vi "Test All.vi"(11 "Error in":errorcluster) -> (15 "Error out":errorcluster)   [LabVIEW 2020, in "CelsiusToFarenheitTests.lvlib"]
doc: "This vi runs all the test cases for the Celsius to Fahrenheit assignment. Also the test report gets saved as a xml format.\n\n* USES *\nDrona, G-CLI and Caraya"
uses:
  CelsiusToFarenheitTests.lvlib
  <vilib>/addons/_JKI Toolkits/Caraya/classes/Test Suite/Define Test Suite (JUnit Report).vi
  <vilib>/Utility/error.llb/Error Cluster From Error Code.vi
  <vilib>/ErrorRing/Error Ring.xnode
  <vilib>/addons/_JKI Toolkits/Caraya/classes/Test Suite/Test Suite.lvclass
  <vilib>/addons/_JKI Toolkits/Caraya/classes/Test/Test.lvclass
  <vilib>/Wiresmith Technology/G CLI/CLI Class/CLI.lvclass
panel:
  # "TESTING ALL TEST CASES FOR CELSIUS TO FAHRENHEIT"
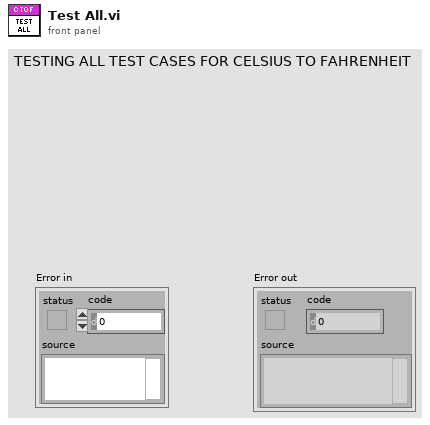
[diagram p1: front panel]
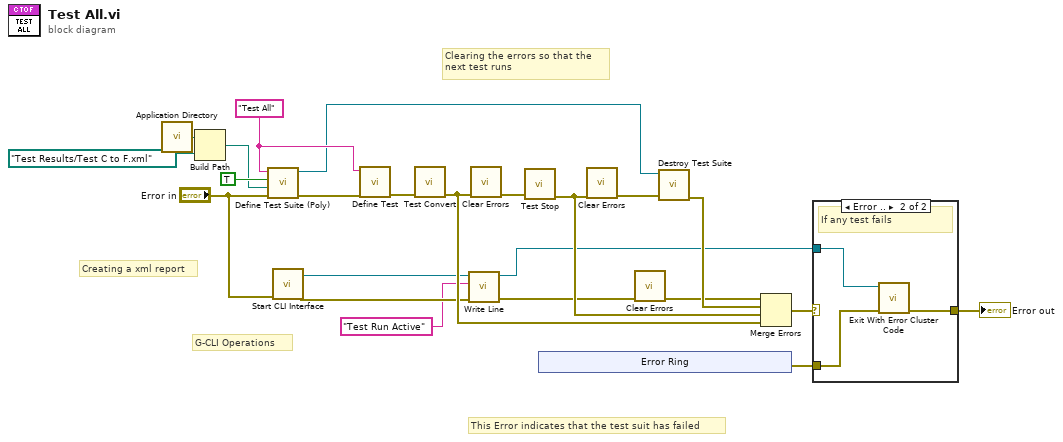
[diagram p0: block diagram]
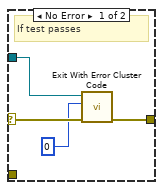
[diagram p2: hidden frame]
diagram:
  w18 = "Test All" ("Label (VI Title)")
  # "This Error indicates that the test suit has failed"
  # "G-CLI Operations"
  # "Creating a xml report"
  # "Clearing the errors so that the\nnext test runs"
  n1 = call <vilib>:"Application Directory.vi"() -> ("Application Directory"=w23:path)
  n2 = Build Path(base path=w23, name or relative path=path "Test Results/Test C to F.xml") -> (appended path=w20:path)
  n3 = call-poly <vilib>:"Define Test Suite (Poly).vi"("error in (no error)"="Error in", "Report Path"=w20, "Interactive"=TRUE, "Label (VI Title)"=w18) -> ("error out"=w19:errorcluster, "Test Suite"=w17:refnum<class "Test Suite.lvclass">)  [unwired: 6 in]
  n4 = call <vilib>:"Start CLI Interface.vi"("error in (no error)"="Error in") -> ("error out"=w10:errorcluster, "CLI out"=w8:refnum<class "CLI.lvclass">)  [unwired: 7 in, 2 out]
  n5 = call <vilib>:"Define Test.vi"("error in (no error)"=w19, "Label (VI Title)"=w18) -> ("error out"=w16:errorcluster)  [unwired: 9 in]
  n6 = call "Test Convert.vi"("Error in"=w16) -> ("Error out"=w13:errorcluster)  [unwired: 14 in]
  n7 = call <vilib>:"Write Line.vi"("error in (no error)"=w10, "Text to Write"="Test Run Active", "CLI in"=w8) -> ("error out"=w6:errorcluster, "CLI out"=w3:refnum<class "CLI.lvclass">)  [unwired: 7 in]
  n8 = call <vilib>:"Clear Errors.vi"("error in (no error)"=w13) -> ("error out"=w15:errorcluster)  [unwired: 5 in, 1 out]
  n9 = call "Test Stop.vi"("Error in"=w15) -> ("Error out"=w12:errorcluster)  [unwired: 14 in]
  n10 = xnode "Error Ring"() -> ("error out"=w1:errorcluster)
  n11 = call <vilib>:"Clear Errors.vi"("error in (no error)"=w12) -> ("error out"=w14:errorcluster)  [unwired: 5 in, 1 out]
  n12 = call <vilib>:"Clear Errors.vi"("error in (no error)"=w6) -> ("error out"=w5:errorcluster)  [unwired: 5 in, 1 out]
  n13 = call-dynamic "Destroy Test Suite.vi"("error in (no error)"=w14, "Test Suite in"=w17) -> ("error out"=w7:errorcluster)  [unwired: 8 in, 1 out]
  n14 = Merge Errors(w5, w7, w12, w13) -> (w4:errorcluster)
  n15 = case shown="Error .." w4 {
    selector: w4 -> [w27 _]
    tunnel: w3 -> [w26 w28]
    tunnel: [w24 w30] -> w2
    tunnel: w1 -> [_ w29]
    frame No Error {
      # "If test passes"
      n16 = call <vilib>:"Exit With Error Cluster Code.vi"("error in (no error)"=w27, "No Error Code (0)"=0, "CLI in"=w26) -> ("error out"=w24:errorcluster)  [unwired: 8 in]
    }
    frame Error {
      # "If any test fails"
      n17 = call <vilib>:"Exit With Error Cluster Code.vi"("error in (no error)"=w29, "CLI in"=w28) -> ("error out"=w30:errorcluster)  [unwired: 9 in]
    }
  }
  "Error out" <- w2
